vi "Reference Global.vi"() -> ()   [LabVIEW 2013]
panel:
  out "Lookup Table":string[][](table)
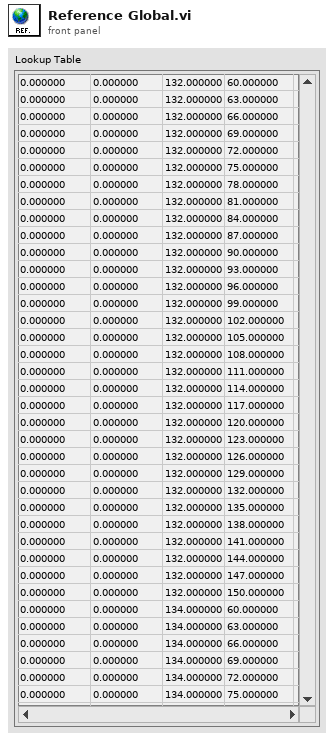
[diagram p1: front panel]
diagram:
